vi "draw a line -- merge.vi"(10 "Array":cluster{dbl[], dbl[]}[](array[cluster])) -> (3 "output cluster":cluster{dbl[], dbl[]})   [LabVIEW 2018]
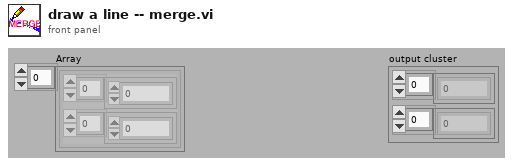
[diagram p1: front panel]
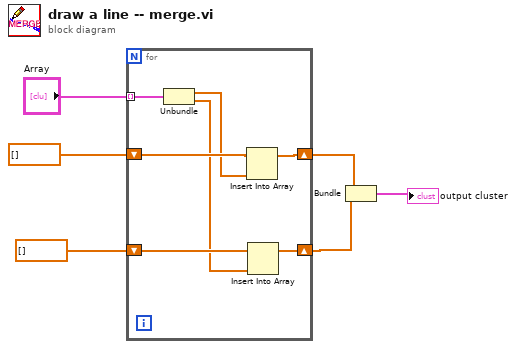
[diagram p0: block diagram]
diagram:
  n1 = for {
    tunnel: "Array" -> [w13] mode=indexing
    shift-right: [w9] -> w3
    shift-left: dbl[] [] -> [w10]
    shift-right: [w11] -> w2
    shift-left: dbl[] [] -> [w12]
    n2 = Unbundle(w13) -> (w8:dbl[], w7:dbl[])
    n3 = Insert Into Array(array=w10, new element=w8) -> (w9:dbl[])  [unwired: 1 in]
    n4 = Insert Into Array(array=w12, new element=w7) -> (w11:dbl[])  [unwired: 1 in]
  }
  n5 = Bundle(w3, w2) -> (→"output cluster":cluster{dbl[], dbl[]})  [unwired: 1 in]
